vi "binary_get_calibration_coefficients.vi"(8 "error in":errorcluster, 9 "calibrations?":bool, 10 "all in one package input":T1={"memory structure"={"length of metadata [byte]"=5, "length of page [byte]"=2048, "length of measurement data on page [byte]"=2028, "length of dataset [byte]"=6}, "actigraph settings"={"sampling frequency [Hz]"=0.0, "measurement interval [± g]"=0, "high precision?"=FALSE, "number of pages"=0, "rate code"=0, "range code"=0, "id"=0}, "time informations"={"starting time"=timestamp(0 s since 1904-01-01), "ending time"=timestamp(0 s since 1904-01-01), "dt[s]"=0.0, "sampling rate [Hz]"=0.0, "length"=0.0}, "measurement data"={"number of samples per axis"=0, "timestamp array"=[], "offset array"=[], "x, y, z axis data"=[], "normalised magnitude of acceleartion vectors"={"t0"=timestamp(0 s since 1904-01-01), "dt"=1.0, "Y"=[]}, "calibration coefficients"={"Sx"=0.0, "Ox"=0.0, "Sy"=0.0, "Oy"=0.0, "Sz"=0.0, "Oz"=0.0}, "statistics"={"mean of x axis acceleration"=0.0, "standard devation of x axis acceleration"=0.0, "mean of y axis acceleration"=0.0, "standard devation of y axis acceleration"=0.0, "mean of z axis acceleration"=0.0, "standard devation of z axis acceleration"=0.0, "mean of normalised magnitude of acceleration"=0.0, "standard devation of normalised magnitude of acceleration"=0.0}, "battery voltage"={"t0"=timestamp(0 s since 1904-01-01), "dt"=1.0, "Y"=[]}, "magnitude of acceleartion vectors"={"t0"=timestamp(0 s since 1904-01-01), "dt"=1.0, "Y"=[]}}} {"measurement data"."calibration coefficients"."Oz" format="%#_12g"; "measurement data"."calibration coefficients"."Sz" format="%#_12g"; "measurement data"."calibration coefficients"."Oy" format="%#_12g"; "measurement data"."calibration coefficients"."Sy" format="%#_12g"; "measurement data"."calibration coefficients"."Ox" format="%#_12g"; "measurement data"."calibration coefficients"."Sx" format="%#_12g"; "time informations"."length" format="%<%H:%M:%S%3u>t"; "actigraph settings"."id" format="%02d"; "actigraph settings"."range code" format="%02x"; "actigraph settings"."rate code" format="%02x"}, 11 "binary data":u8[](array[numeric])) -> (0 "error out":errorcluster, 2 "all in one package output":T1={"memory structure"={"length of metadata [byte]"=5, "length of page [byte]"=2048, "length of measurement data on page [byte]"=2028, "length of dataset [byte]"=6}, "actigraph settings"={"sampling frequency [Hz]"=0.0, "measurement interval [± g]"=0, "high precision?"=FALSE, "number of pages"=0, "rate code"=0, "range code"=0, "id"=0}, "time informations"={"starting time"=timestamp(0 s since 1904-01-01), "ending time"=timestamp(0 s since 1904-01-01), "dt[s]"=0.0, "sampling rate [Hz]"=0.0, "length"=0.0}, "measurement data"={"number of samples per axis"=0, "timestamp array"=[], "offset array"=[], "x, y, z axis data"=[], "normalised magnitude of acceleartion vectors"={"t0"=timestamp(0 s since 1904-01-01), "dt"=1.0, "Y"=[]}, "calibration coefficients"={"Sx"=0.0, "Ox"=0.0, "Sy"=0.0, "Oy"=0.0, "Sz"=0.0, "Oz"=0.0}, "statistics"={"mean of x axis acceleration"=0.0, "standard devation of x axis acceleration"=0.0, "mean of y axis acceleration"=0.0, "standard devation of y axis acceleration"=0.0, "mean of z axis acceleration"=0.0, "standard devation of z axis acceleration"=0.0, "mean of normalised magnitude of acceleration"=0.0, "standard devation of normalised magnitude of acceleration"=0.0}, "battery voltage"={"t0"=timestamp(0 s since 1904-01-01), "dt"=1.0, "Y"=[]}, "magnitude of acceleartion vectors"={"t0"=timestamp(0 s since 1904-01-01), "dt"=1.0, "Y"=[]}}} {"measurement data"."calibration coefficients"."Oz" format="%#_12g"; "measurement data"."calibration coefficients"."Sz" format="%#_12g"; "measurement data"."calibration coefficients"."Oy" format="%#_12g"; "measurement data"."calibration coefficients"."Sy" format="%#_12g"; "measurement data"."calibration coefficients"."Ox" format="%#_12g"; "measurement data"."calibration coefficients"."Sx" format="%#_12g"; "time informations"."length" format="%<%H:%M:%S%3u>t"; "actigraph settings"."id" format="%02d"; "actigraph settings"."range code" format="%02x"; "actigraph settings"."rate code" format="%02x"}, 3 "binary data w/ calibration coefficients":u8[](array[numeric]))   [LabVIEW 2017]
uses:
  Controls/control_all_in_one_package.ctl
  Controls/control_memory_structure.ctl
  Controls/control_measurement_settings.ctl
  Controls/control_time_informations.ctl
  Controls/control_measurement_data.ctl
  Controls/control_calibration_coefficients.ctl
  Controls/control_statistics.ctl
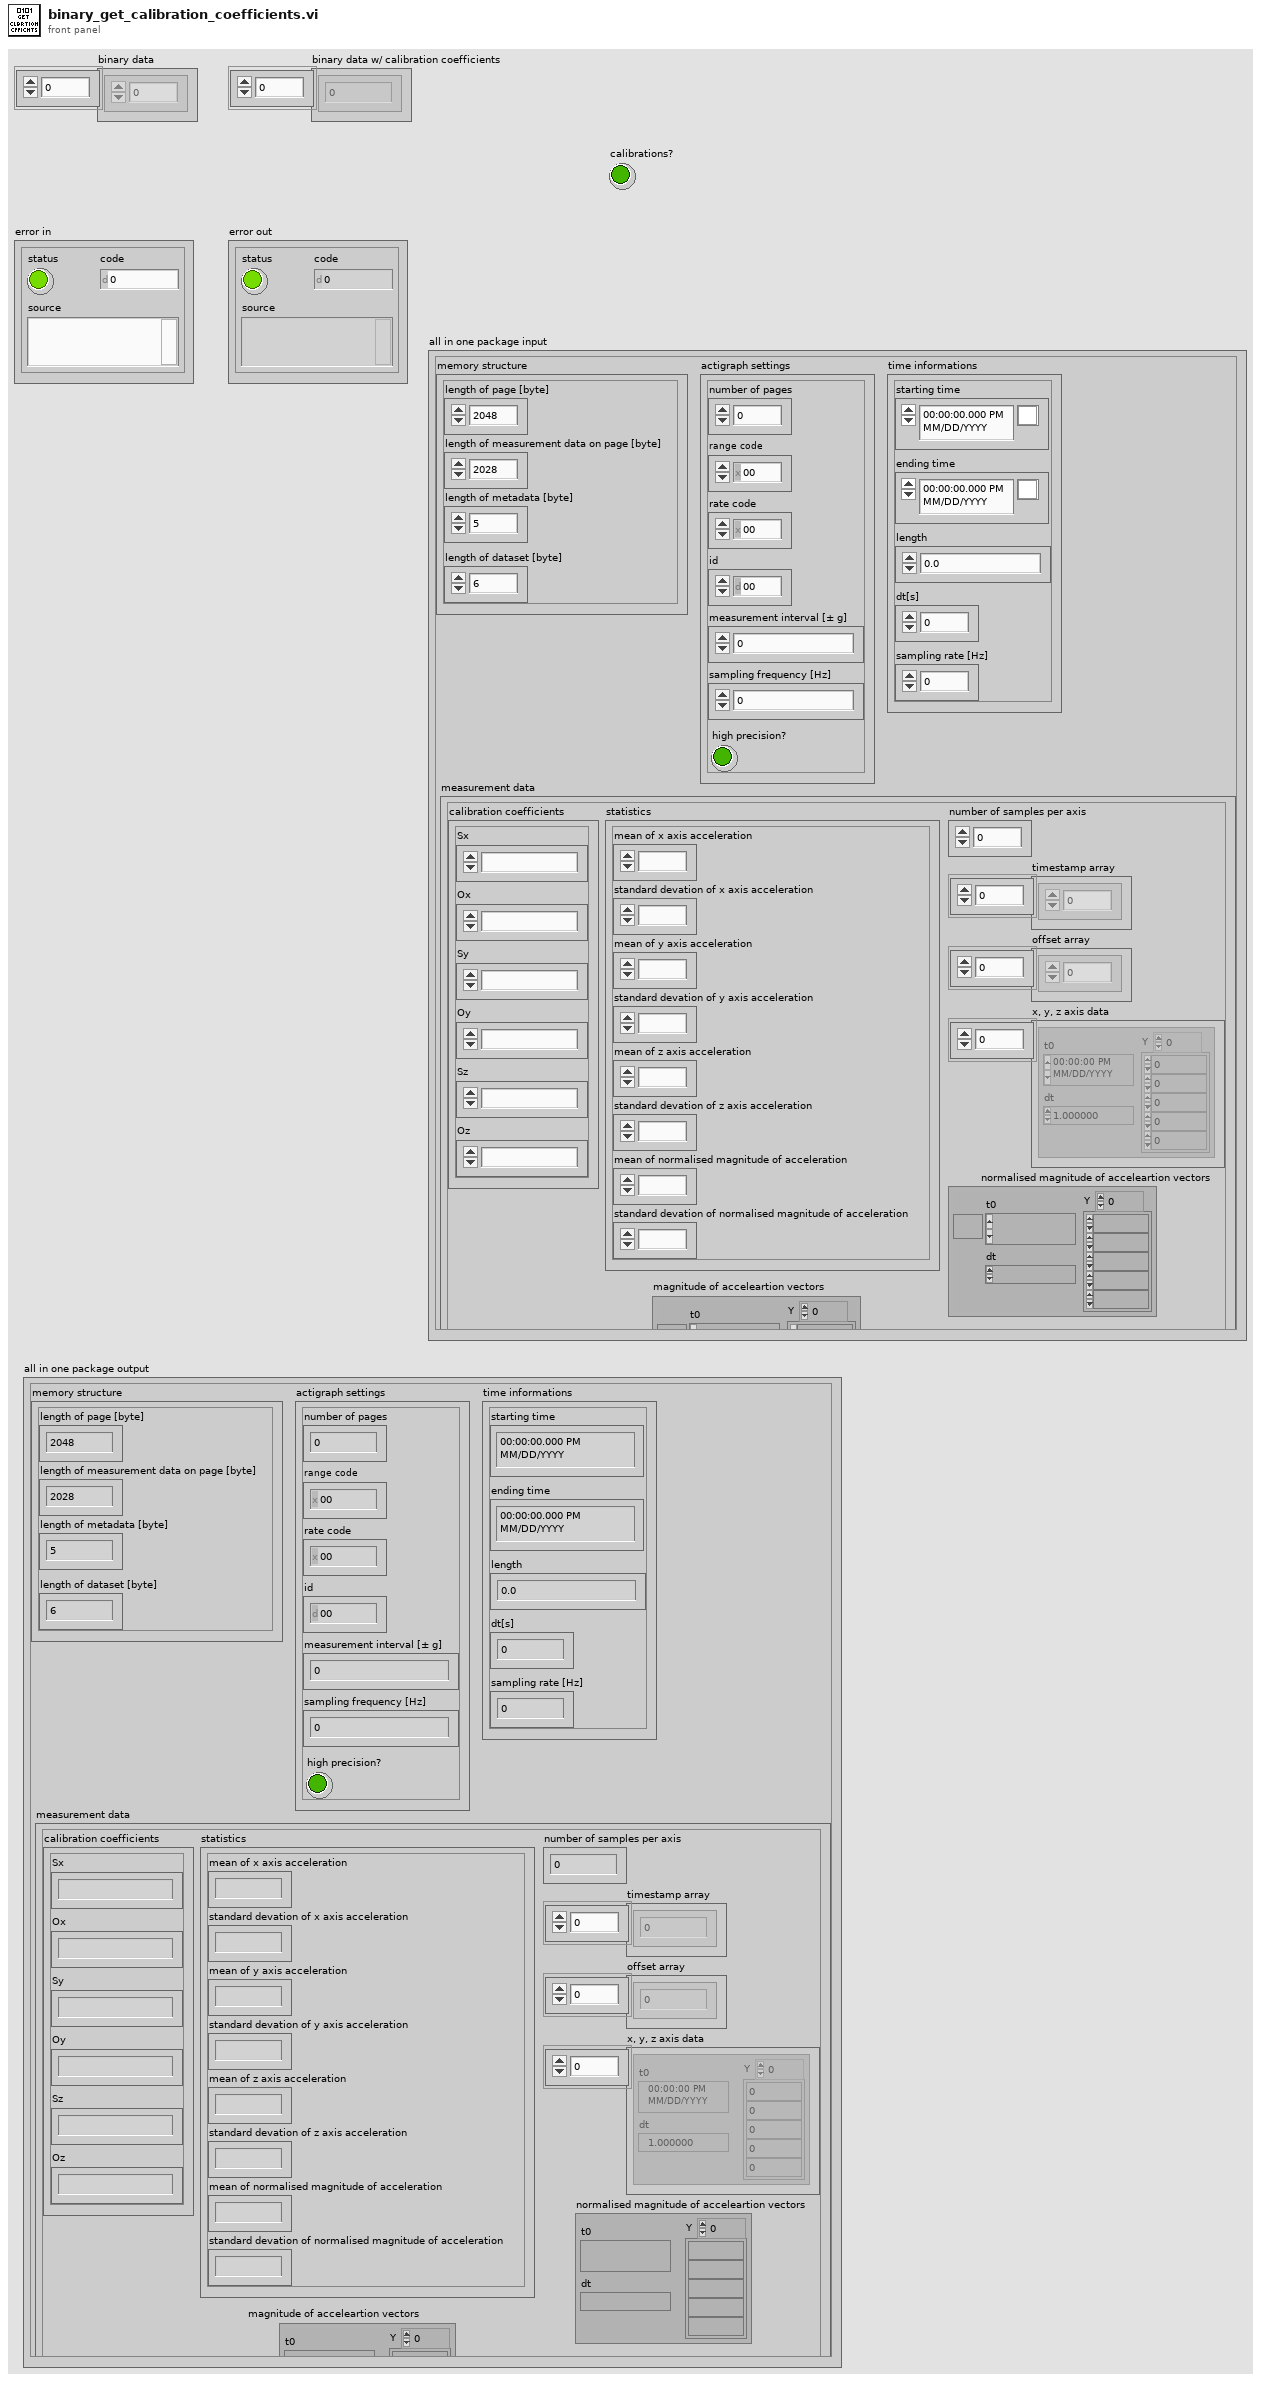
[diagram p1: front panel]
types:
  T1 = typedef "control_all_in_one_package.ctl" = cluster{"memory structure":T2, "actigraph settings":T3, "time informations":T4, "measurement data":T5}
  T2 = typedef "control_memory_structure.ctl" = cluster{"length of metadata [byte]":i32, "length of page [byte]":i32, "length of measurement data on page [byte]":i32, "length of dataset [byte]":i32}
  T3 = typedef "control_measurement_settings.ctl" = cluster{"sampling frequency [Hz]":dbl, "measurement interval [± g]":i32, "high precision?":bool, "number of pages":i32, "rate code":i32, "range code":i32, "id":i32}
  T4 = typedef "control_time_informations.ctl" = cluster{"starting time":timestamp, "ending time":timestamp, "dt[s]":dbl, "sampling rate [Hz]":dbl, "length":dbl}
  T5 = typedef "control_measurement_data.ctl" = cluster{"number of samples per axis":i32, "timestamp array":dbl[], "offset array":dbl[], "x, y, z axis data":waveform(dbl)[], "normalised magnitude of acceleartion vectors":waveform(dbl), "calibration coefficients":T6, "statistics":T7, "battery voltage":waveform(dbl), "magnitude of acceleartion vectors":waveform(dbl)}
  T6 = typedef "control_calibration_coefficients.ctl" = cluster{"Sx":dbl, "Ox":dbl, "Sy":dbl, "Oy":dbl, "Sz":dbl, "Oz":dbl}
  T7 = typedef "control_statistics.ctl" = cluster{"mean of x axis acceleration":dbl, "standard devation of x axis acceleration":dbl, "mean of y axis acceleration":dbl, "standard devation of y axis acceleration":dbl, "mean of z axis acceleration":dbl, "standard devation of z axis acceleration":dbl, "mean of normalised magnitude of acceleration":dbl, "standard devation of normalised magnitude of acceleration":dbl}
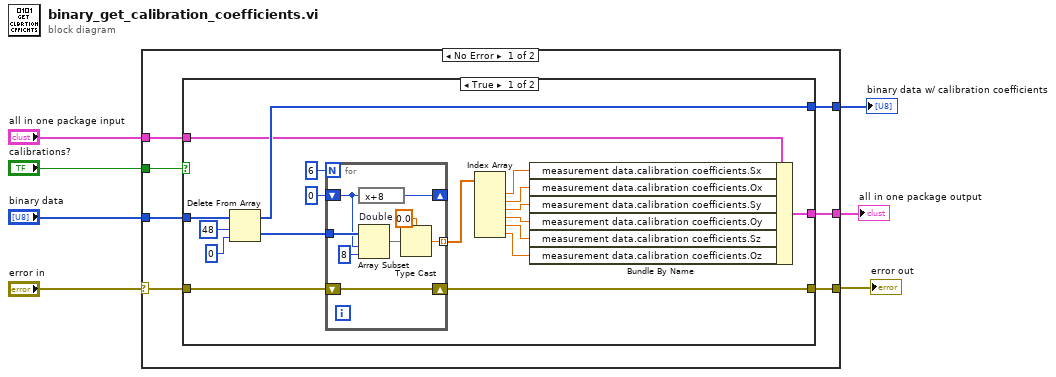
[diagram p0: block diagram]
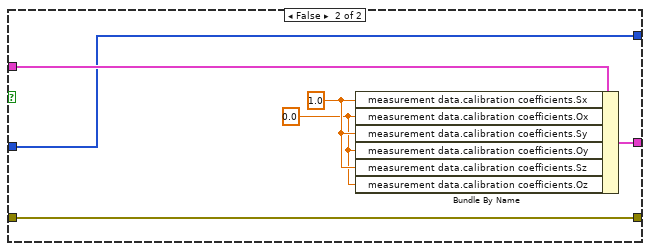
[diagram p2: hidden frame]
diagram:
  n1 = case shown="No Error" "error in" {
    selector: "error in" -> [w9 w49]
    tunnel: "binary data" -> [w14 w47]
    tunnel: [w13 w49] -> w2
    tunnel: [w12 w47] -> w6
    tunnel: "all in one package input" -> [w11 w48]
    tunnel: [w10 w48] -> w4
    tunnel: "calibrations?" -> [w8 _]
    frame No Error {
      n2 = case shown="True" w8 {
        tunnel: w14 -> [w29 w43]
        tunnel: [w28 w44] -> w13
        tunnel: [w27 w43] -> w12
        tunnel: w11 -> [w24 w46]
        tunnel: [w16 w45] -> w10
        tunnel: w9 -> [w15 w44]
        frame True {
          n3 = Delete From Array(array=w29, length=48 ("index"), index=0 ("length")) -> (deleted portion=w32:u8[], array with subset deleted=w27:u8[])
          n4 = for {
            N: 6 -> [_]
            shift-right: [w40] -> _
            shift-left: 0 ("offset (in bytes) (0)") -> [w38]
            tunnel: w32 -> [w39]
            tunnel: [w34] -> w23 mode=indexing
            shift-right: [w33] -> w28
            shift-left: w15 -> [w33]
            w36 = 0.0  # Double
            n5 = expression code="x+8"(w38) -> (w40:i32)
            n6 = Array Subset(array=w39, index=w38, length=8) -> (w35:u8[])
            n7 = Type Cast(type=w36, x=w35) -> (*(type *) &x=w34:dbl)
          }
          n8 = Index Array(array=w23) -> (element #1=w17:dbl, element #2=w20:dbl, element #3=w22:dbl, element #4=w21:dbl, element #5=w19:dbl, element #6=w18:dbl)  [unwired: 6 in]
          n9 = Bundle By Name(cluster=w24, "measurement data.calibration coefficients.Sx"=w17, "measurement data.calibration coefficients.Ox"=w20, "measurement data.calibration coefficients.Sy"=w22, "measurement data.calibration coefficients.Oy"=w21, "measurement data.calibration coefficients.Sz"=w19, "measurement data.calibration coefficients.Oz"=w18) -> (w16:T1)
        }
        frame False {
          w41 = 0.0 ("measurement data.Calibration coefficients.Sx")
          w42 = 1.0 ("measurement data.Calibration coefficients.Sx")
          n10 = Bundle By Name(cluster=w46, "measurement data.calibration coefficients.Sx"=w42, "measurement data.calibration coefficients.Ox"=w41, "measurement data.calibration coefficients.Sy"=w42, "measurement data.calibration coefficients.Oy"=w41, "measurement data.calibration coefficients.Sz"=w42, "measurement data.calibration coefficients.Oz"=w41) -> (w45:T1)
        }
      }
    }
    frame Error {
    }
  }
  "error out" <- w2
  "binary data w/ calibration coefficients" <- w6
  "all in one package output" <- w4
